vi "Energy (N Channels).vi"(7 "reset? (F)":bool, 8 "error in (no error)":errorcluster, 9 "start timestamp":timestamp, 10 "interval length [s]":dbl=0.2, 11 "power values":T1[](array[typedef])) -> (0 "error out":errorcluster, 1 "measurement timestamps":T3, 3 "energy values":T2[](array[typedef]))   [LabVIEW 2014, in "NI_EP_Basic.lvlib"]
doc: "Calculates the energy value from the power value for a specified interval. This VI returns the value of active energy, apparent energy, and reactive energy. Wire data to the <B>power value</B> input to determine the polymorphic instance to use or manually select the instance."
uses:
  <vilib>/addons/Electrical Power/Basic/NI_EP_Basic.lvlib
  <vilib>/addons/Electrical Power/Basic/Measurement/subVIs/basic_Energy Value.ctl
  <vilib>/addons/Electrical Power/Basic/Measurement/subVIs/basic_Power Value.ctl
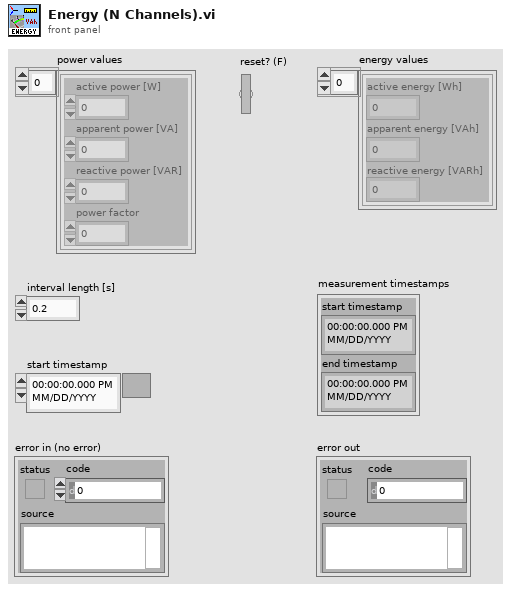
[diagram p1: front panel]
types:
  T1 = typedef "NI_EP_Basic.lvlib/basic_Power Value.ctl" = cluster{"active power [W]":dbl, "apparent power [VA]":dbl, "reactive power [VAR]":dbl, "power factor":dbl}
  T2 = typedef "NI_EP_Basic.lvlib/basic_Energy Value.ctl" = cluster{"active energy [Wh]":dbl, "apparent energy [VAh]":dbl, "reactive energy [VARh]":dbl}
  T3 = cluster{"start timestamp":timestamp, "end timestamp":timestamp}
  T4 = cluster{"start time stamp":timestamp, "end time stamp":timestamp}
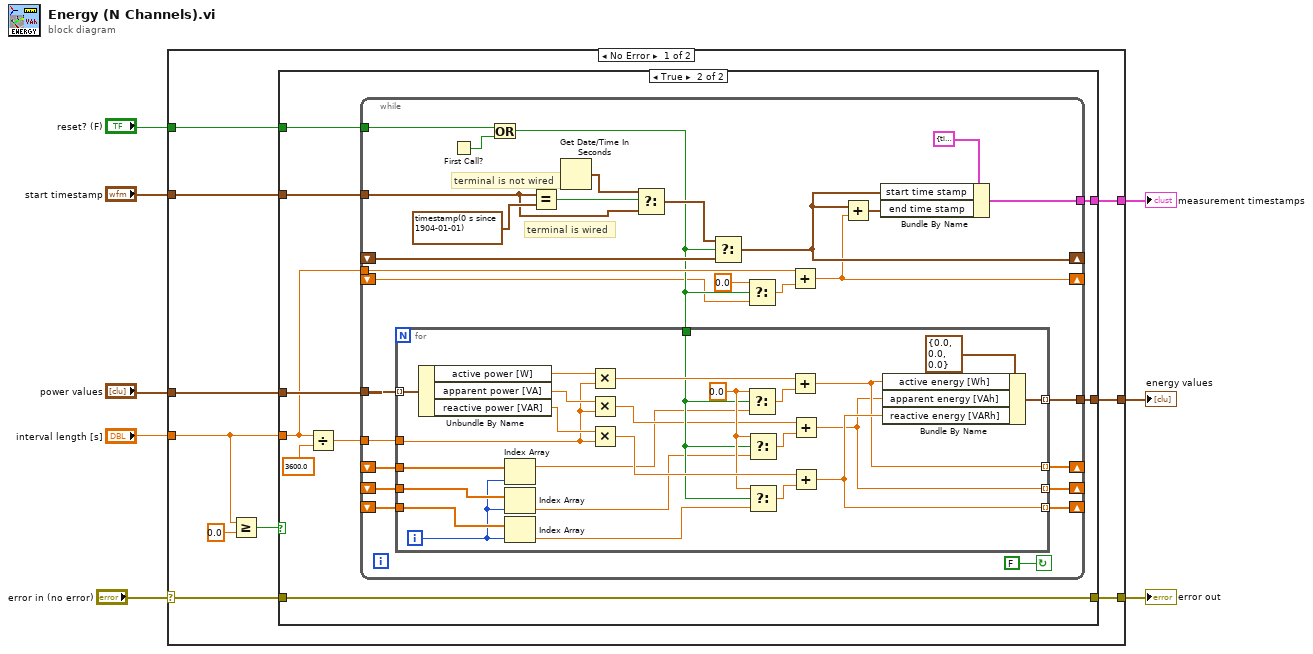
[diagram p0: block diagram]
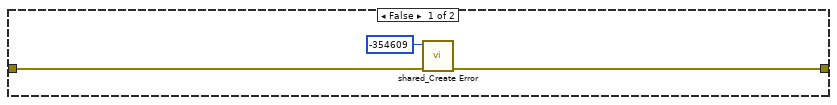
[diagram p2: hidden frame]
diagram:
  n1 = case shown="No Error" "error in (no error)" {
    selector: "error in (no error)" -> [w9 w84]
    tunnel: "reset? (F)" -> [w18 _]
    tunnel: "start timestamp" -> [w17 _]
    tunnel: [w16 _] -> w6
    tunnel: [w15 _] -> w5
    tunnel: "power values" -> [w14 _]
    tunnel: "interval length [s]" -> [w11 _]
    tunnel: [w10 w84] -> w1
    frame No Error {
      n2 = Greater Or Equal?(x=w11, y=0.0) -> (x >= y?=w12:bool)
      n3 = case shown="True" w12 {
        tunnel: w18 -> [_ w30]
        tunnel: w17 -> [_ w29]
        tunnel: [_ w26] -> w16
        tunnel: [_ w25] -> w15
        tunnel: w14 -> [_ w24]
        tunnel: w11 -> [_ w23]
        tunnel: [w19 w22] -> w10
        tunnel: w9 -> [w20 w22]
        frame False {
          n4 = call <vilib>:"shared_Create Error.vi"("error in (no error)"=w20, "error code (0)"=-354609) -> ("error out"=w19:errorcluster)  [unwired: 9 in]
        }
        frame True {
          n5 = Divide(x=w23, y=3600.0) -> (x/y=w27:dbl)
          n6 = while {
            tunnel: w24 -> [w58]
            tunnel: w30 -> [w56]
            tunnel: w29 -> [w52]
            tunnel: w27 -> [w44]
            tunnel: [w50] -> w25
            tunnel: [w49] -> w26
            shift-right: [w39] -> _
            shift-left: _ -> [w40]
            shift-right: [w41] -> _
            shift-left: _ -> [w42]
            shift-right: [w31] -> _
            shift-left: _ -> [w43]
            shift-right: [w32] -> _
            shift-left: _ -> [w33]
            shift-right: [w46] -> _
            shift-left: _ -> [w45]
            tunnel: w23 -> [w35]
            stop <- FALSE continue-if-true
            # "terminal is wired"
            # "terminal is not wired"
            n7 = First Call?() -> (First Call?: T/F=w57:bool)
            n8 = Or(x=w56, y=w57) -> (x .or. y?=w34:bool)
            n9 = for {
              tunnel: w58 -> [w83] mode=indexing
              tunnel: [w79] -> w49 mode=indexing
              tunnel: w34 -> [w68]
              tunnel: w44 -> [w77]
              tunnel: w40 -> [w61]
              tunnel: [w74] -> w39 mode=indexing
              tunnel: w43 -> [w65]
              tunnel: [w72] -> w31 mode=indexing
              tunnel: w42 -> [w63]
              tunnel: [w67] -> w41 mode=indexing
              i -> [w59]
              w69 = 0.0 ("t")
              n10 = Unbundle By Name(w83) -> ("active power [W]"=w82:dbl, "apparent power [VA]"=w78:dbl, "reactive power [VAR]"=w81:dbl)
              n11 = Index Array(array=w65, index=w59) -> (element=w64:dbl)
              n12 = Index Array(array=w63, index=w59) -> (element=w62:dbl)
              n13 = Index Array(array=w61, index=w59) -> (element=w60:dbl)
              n14 = Multiply(x=w82, y=w77) -> (x*y=w70:dbl)
              n15 = Multiply(x=w78, y=w77) -> (x*y=w66:dbl)
              n16 = Multiply(x=w81, y=w77) -> (x*y=w75:dbl)
              n17 = Select(t=w69, s=w68, f=w64) -> (s? t:f=w73:dbl)
              n18 = Select(t=w69, s=w68, f=w62) -> (s? t:f=w71:dbl)
              n19 = Select(t=w69, s=w68, f=w60) -> (s? t:f=w76:dbl)
              n20 = Add(x=w70, y=w73) -> (x+y=w72:dbl)
              n21 = Add(x=w66, y=w71) -> (x+y=w67:dbl)
              n22 = Add(x=w75, y=w76) -> (x+y=w74:dbl)
              n23 = Bundle By Name(cluster=T2 {"active energy [Wh]"=0.0, "apparent energy [VAh]"=0.0, "reactive energy [VARh]"=0.0} ("energy  value"), "active energy [Wh]"=w72, "apparent energy [VAh]"=w67, "reactive energy [VARh]"=w74) -> (w79:T2)
            }
            n24 = Equal?(x=w52, y=timestamp(0 s since 1904-01-01) ("time stamp")) -> (x = y?=w53:bool)
            n25 = Get Date/Time In Seconds() -> (seconds since 1Jan1904=w55:timestamp)
            n26 = Select(t=w55, s=w53, f=w52) -> (s? t:f=w47:timestamp)
            n27 = Select(t=w47, s=w34, f=w45) -> (s? t:f=w46:timestamp)
            n28 = Select(t=0.0, s=w34, f=w33) -> (s? t:f=w37:dbl)
            n29 = Add(x=w35, y=w37) -> (x+y=w32:dbl)
            n30 = Add(x=w46, y=w32) -> (x+y=w38:timestamp)
            n31 = Bundle By Name(cluster=T4 {"start time stamp"=timestamp(0 s since 1904-01-01), "end time stamp"=timestamp(0 s since 1904-01-01)} ("measurement time stamps"), "start time stamp"=w46, "end time stamp"=w38) -> (w50:T4)
          }
        }
      }
    }
    frame Error {
    }
  }
  "measurement timestamps" <- w5
  "error out" <- w1
  "energy values" <- w6
